vi "Ini RFID ftdi.vi"(10 "Power":u32=500 max=2700 step=10, 11 "COM RFID":refnum<visa-resource-name>="COM4") -> (0 "Err Out":errorcluster, 2 "WR Str":string, 3 "Ini ?":bool)   [LabVIEW 2018]
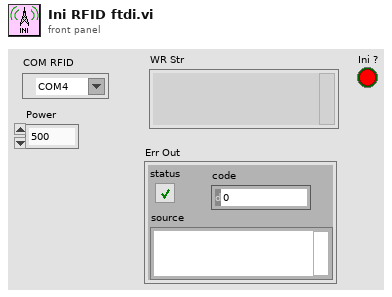
[diagram p1: front panel]
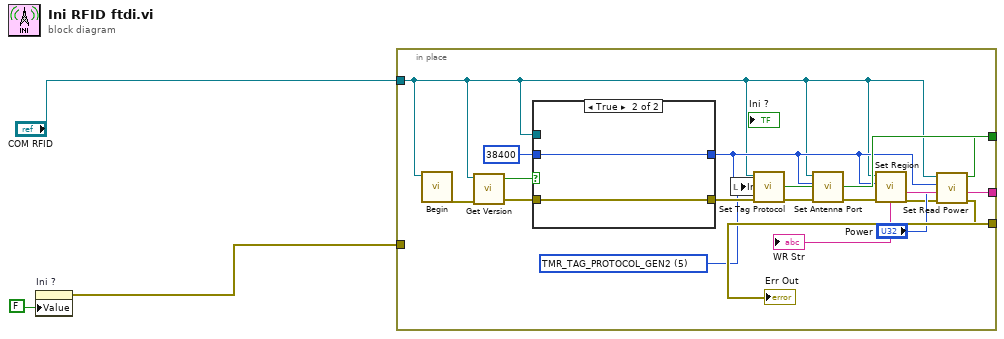
[diagram p0: block diagram]
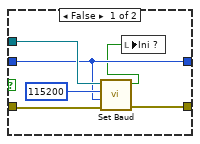
[diagram p2: hidden frame]
diagram:
  n1 = property on="Ini ?" class="Bool (strict)"("Value"=FALSE ("Ini ?")) -> (error out=w1:errorcluster)  [unwired: 2 in, 1 out]
  n2 = in-place {
    in-place-border: [w16] -> w6
    in-place-border: [w15] -> w5
    in-place-border: "COM RFID" -> [w8]
    in-place-border: [w7] -> w3
    in-place-border: w1 -> [_]
    w10 = u16 5 items=["TMR_TAG_PROTOCOL_NONE"=0, "TMR_TAG_PROTOCOL_ISO180006B"=3, "TMR_TAG_PROTOCOL_GEN2"=5, "TMR_TAG_PROTOCOL_ISO180006B_UCODE"=6, "TMR_TAG_PROTOCOL_IPX64"=7, "TMR_TAG_PROTOCOL_IPX256"=8, "TMR_TAG_PROTOCOL_ATA"=29] ("Tag Protocol")
    n3 = call "Begin.vi"("COM Port"=w8) -> ("error out"=w18:errorcluster)  [unwired: 10 in]
    n4 = call "Get Version.vi"("error in (no error)"=w18, "COM Port"=w8) -> ("error out"=w19:errorcluster, "Result"=w20:bool)  [unwired: 7 in, 1 out]
    n5 = case shown="True" w20 {
      tunnel: [w26 w29] -> w17
      tunnel: [w23 w28] -> w9
      tunnel: w19 -> [w25 w29]
      tunnel: w8 -> [w24 _]
      tunnel: u32 38400 ("New Baud") -> [w23 w28]
      frame False {
        n6 = call "Set Baud.vi"("error in (no error)"=w25, "New Baud"=w23, "Old Baud"=u32 115200, "COM Port"=w24) -> ("error out"=w26:errorcluster, "Result"=w22:bool)  [unwired: 6 in]
        n7 = local write "Ini ?"(w22) -> ()
      }
      frame True {
      }
    }
    n8 = call "Set Tag Protocol.vi"("error in (no error)"=w17, "Protocol"=w10, "Baud Rate"=w9, "COM Port"=w8) -> ("error out"=w11:errorcluster)  [unwired: 5 in, 2 out]
    n9 = call "Set Antenna Port.vi"("error in (no error)"=w11, "Baud Rate"=w9, "COM Port"=w8) -> ("error out"=w12:errorcluster)  [unwired: 6 in, 2 out]
    n10 = call "Set Region.vi"("error in (no error)"=w12, "Baud Rate"=w9, "COM Port"=w8) -> ("error out"=w13:errorcluster)  [unwired: 6 in, 2 out]
    n11 = call "Set Read Power.vi"("error in (no error)"=w13, "Power"="Power", "Baud"=w9, "COM Port"=w8) -> ("error out"=w16:errorcluster, "received str"=w15:string, "Result"=w7:bool)  [unwired: 5 in]
  }
  "WR Str" <- w5
  "Err Out" <- w6
  n12 = local write "Ini ?"(w3) -> ()
